vi "GEOM_ParsePars.vi"(9 "ref val":dbl, 10 "par in":string) -> (1 "val out":dbl)   [LabVIEW 2016]
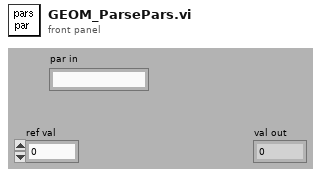
[diagram p1: front panel]
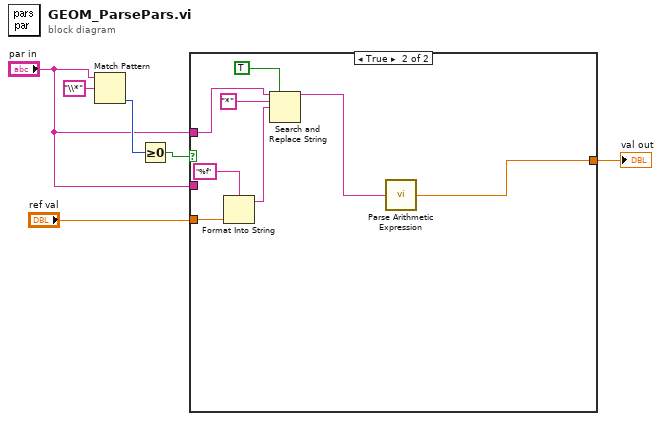
[diagram p0: block diagram]
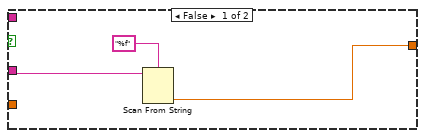
[diagram p2: hidden frame]
diagram:
  n1 = Match Pattern(string="par in", regular expression="\\*") -> (offset past match=w5:i32)  [unwired: 4 out]
  n2 = Greater Or Equal To 0?(x=w5) -> (x >= 0?=w4:bool)
  n3 = case shown="True" w4 {
    tunnel: "ref val" -> [_ w16]
    tunnel: "par in" -> [w9 _]
    tunnel: [w7 w10] -> w2
    tunnel: "par in" -> [_ w13]
    frame False {
      n4 = Scan From String(format string="%f", input string=w9) -> (output 1=w7:dbl)  [unwired: 2 in, 4 out]
    }
    frame True {
      n5 = Format Into String(format string="%f", w16) -> (resulting string=w15:string)  [unwired: 2 in, 1 out]
      n6 = Search and Replace String(replace all?=TRUE ("replace all? (F)"), input string=w13, search string="*", replace string=w15) -> (result string=w12:string)  [unwired: 1 in, 6 out]
      n7 = call "Parse Arithmetic Expression.vi"("Arithmetic Expression"=w12) -> ("Result"=w10:dbl)
    }
  }
  "val out" <- w2
